vi "Write waveform pol.vi"   [LabVIEW 2019]
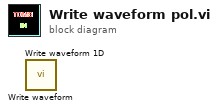
[diagram p0: block diagram]
diagram:
  n1 = call "Write waveform.vi"() -> ()  [unwired: 11 in, 1 out]
  n2 = call "Write waveform 1D.vi"() -> ()  [unwired: 11 in, 1 out]
